vi "Get Control References.vi"(8 "error in (no error)":errorcluster, 9 "Controls to Exclude":refnum<vi>[](array[refnum]), 10 "VI Refnum":refnum<vi>, 11 "AutoRegistration In":refnum<class "AutoRegistration.lvclass">) -> (0 "error out":errorcluster, 2 "Registered":T1, 3 "AutoRegistration Out":refnum<class "AutoRegistration.lvclass">)   [LabVIEW 2015, in "AutoRegistration.lvlib" / "AutoRegistration.lvclass"]
uses:
  AutoRegistration.lvclass
  Registration References.ctl
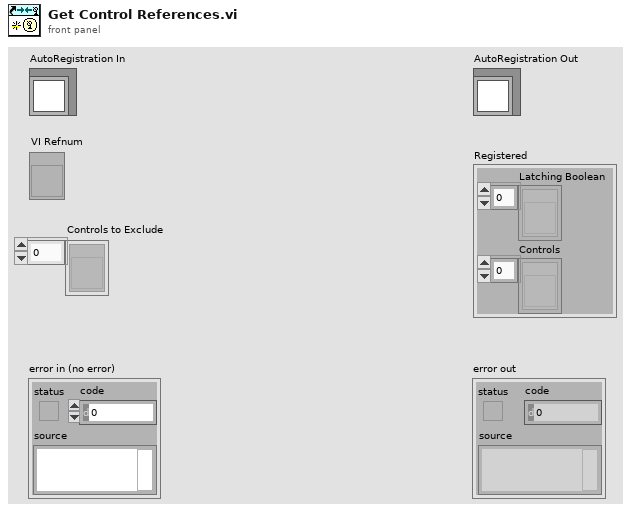
[diagram p1: front panel]
types:
  T1 = typedef "AutoRegistration.lvlib/AutoRegistration.lvclass/Registration References.ctl" = cluster{"Latching Boolean":refnum<vi>[], "Controls":refnum<vi>[]}
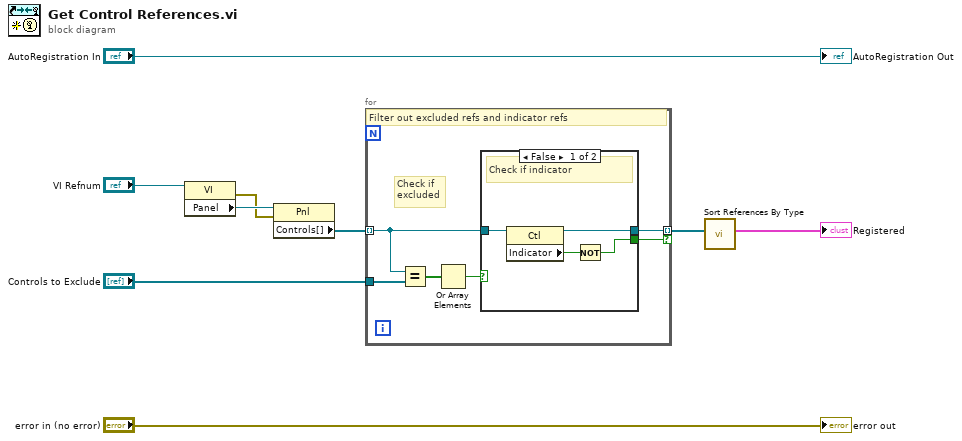
[diagram p0: block diagram]
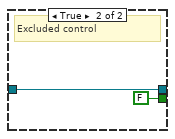
[diagram p2: hidden frame]
diagram:
  n1 = property class="VI"(reference="VI Refnum") -> (error out=w5:errorcluster, "Panel"=w6:refnum<vi>)  [unwired: 1 in, 1 out]
  n2 = property class="Pnl"(reference=w6, error in=w5) -> ("Controls[]"=w4:refnum<vi>[])  [unwired: 2 out]
  n3 = for {
    tunnel: w4 -> [w11] mode=indexing
    tunnel: "Controls to Exclude" -> [w15]
    tunnel: [w10] -> w1 mode=indexing if=w12
    # "Check if\nexcluded"
    # "Filter out excluded refs and indicator refs"
    n4 = Equal?(x=w11, y=w15) -> (x = y?=w14:bool[])
    n5 = Or Array Elements(Boolean array=w14) -> (logical OR=w13:bool)
    n6 = case shown="False" w13 {
      tunnel: [w17 FALSE] -> w12
      tunnel: w11 -> [w19 w20]
      tunnel: [w16 w20] -> w10
      frame False {
        # "Check if indicator"
        n7 = property class="Ctl"(reference=w19) -> (reference out=w16:refnum<vi>, "Indicator"=w18:bool)  [unwired: 1 in, 1 out]
        n8 = Not(x=w18) -> (.not. x?=w17:bool)
      }
      frame True {
        # "Excluded control"
      }
    }
  }
  n9 = call "Sort References By Type.vi"("Controls to Register"=w1) -> ("Controls"=→"Registered":T1)  [unwired: 10 in]
  "error out" <- "error in (no error)"
  "AutoRegistration Out" <- "AutoRegistration In"
